vi "AddMarker.vi"(7 "Time (unconnected for now)":dbl=-999999.0, 8 "error in (no error)":errorcluster, 9 "Description":string, 10 "Label":string, 11 "OXY_SCPI Reseource In":refnum<visa-resource-name>) -> (0 "error out":errorcluster, 1 "communication_data":T1, 3 "OXY_SCPI Reseource IOut":refnum<visa-resource-name>)   [LabVIEW 2018, in "OXYGEN.lvlib"]
doc: "Add markers to current measurement"
uses:
  OXYGEN.lvlib
  TypeDefs/Cluster_RawCommData.ctl
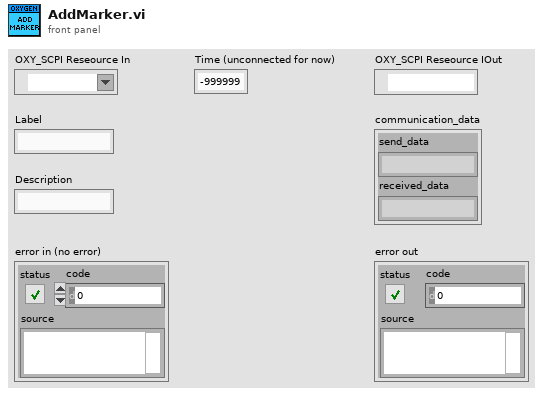
[diagram p1: front panel]
types:
  T1 = typedef "OXYGEN.lvlib/Cluster_RawCommData.ctl" = cluster{"send_data":string, "received_data":string}
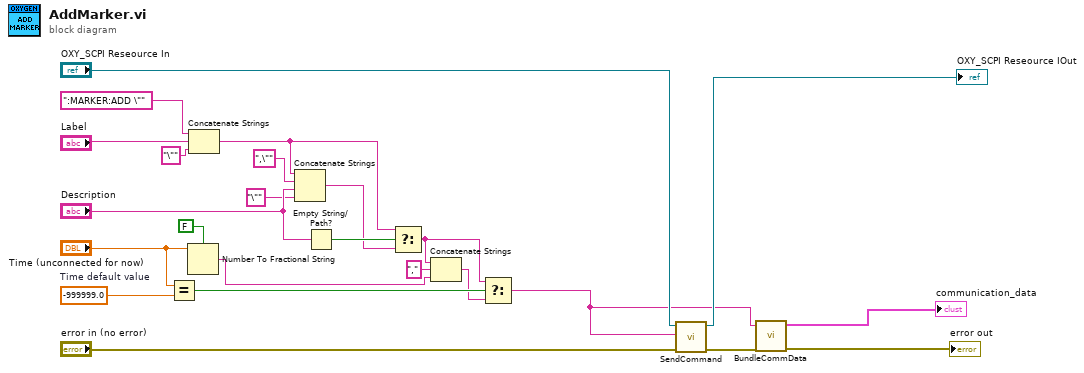
[diagram p0: block diagram]
diagram:
  w18 = -999999.0  # Time default value
  n1 = Equal?(x="Time (unconnected for now)", y=w18) -> (x = y?=w6:bool)
  n2 = Number To Fractional String(use system decimal point (T)=FALSE, number="Time (unconnected for now)") -> (F-format string=w4:string)  [unwired: 2 in]
  n3 = Concatenate Strings(":MARKER:ADD \"" ("string"), "Label", "\"" ("string")) -> (w10:string)
  n4 = Concatenate Strings(w10, ",\"" ("string"), "Description", "\"" ("string")) -> (w11:string)
  n5 = Empty String/Path?(string/path="Description") -> (empty?=w12:bool)
  n6 = Select(t=w10, s=w12, f=w11) -> (s? t:f=w2:string)
  n7 = Concatenate Strings(w2, "," ("string"), w4) -> (w3:string)
  n8 = Select(t=w2, s=w6, f=w3) -> (s? t:f=w1:string)
  n9 = call "SendCommand.vi"("error in (no error)"="error in (no error)", "String to Send"=w1, "OXY_SCPI Reseource In"="OXY_SCPI Reseource In") -> ("error out"=w22:errorcluster, "OXY_SCPI Reseource Out"=→"OXY_SCPI Reseource IOut":refnum<visa-resource-name>)  [unwired: 7 in]
  n10 = call "BundleCommData.vi"("error in (no error)"=w22, "send_data"=w1) -> ("error out"=→"error out":errorcluster, "communication_data"=→"communication_data":T1)  [unwired: 8 in]
